vi "actualizacion de datos.vi"() -> ()   [LabVIEW 2016]
panel:
  out "appended array":dbl[](array[numeric])
  in  "Numeric":dbl
  in  "Array":dbl[](array[numeric])
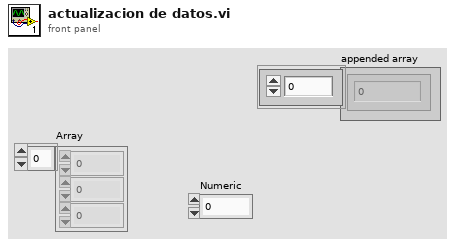
[diagram p1: front panel]
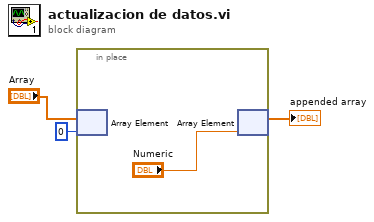
[diagram p0: block diagram]
diagram:
  n1 = in-place {
    n2 = in-place-array #1("Array", 0) -> ()  [unwired: 1 out]
    n3 = in-place-array #1("Numeric") -> (→"appended array":dbl[])  [unwired: 1 out]
  }
